vi "Pre-Build Action.vi"(6 "Top Level/Always Included VIs":path[](array[path]), 7 "Main Destination Path":path, 9 "Target Name":string, 10 "Build Specification Name":string, 11 "Project Path":path) -> (0 "error out":errorcluster)   [LabVIEW 2024]
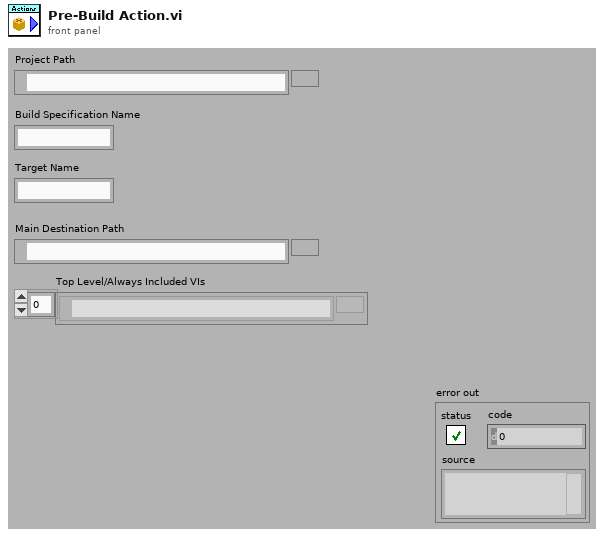
[diagram p1: front panel]
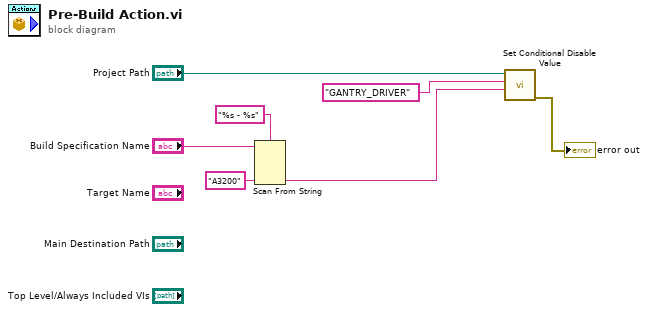
[diagram p0: block diagram]
diagram:
  n1 = Scan From String(format string="%s - %s", input string="Build Specification Name", default 2="A3200" ("default value 2")) -> (output 2=w2:string)  [unwired: 4 in, 3 out]
  n2 = call "Set Conditional Disable Value.vi"("Value"=w2, "Key"="GANTRY_DRIVER" ("Tag Name"), "Project Path"="Project Path") -> ("error out"=→"error out":errorcluster)  [unwired: 8 in]
